vi "CVT Bool GetIndex.vi"(8 "error in (no error)":errorcluster, 11 "Tag Name":string) -> (0 "error out":errorcluster, 3 "Tag Index":i32)   [LabVIEW 2010]
uses:
  Current Value Table.lvlib
  DataTypes/Boolean_Get Index.vi
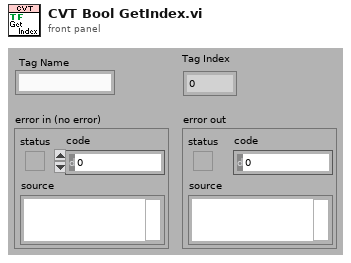
[diagram p1: front panel]
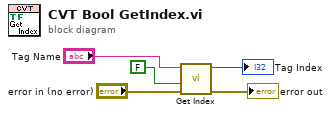
[diagram p0: block diagram]
diagram:
  n1 = call-poly "Get Index.vi"("error in (no error)"="error in (no error)", "Default"=FALSE ("Data Type"), "Tag Name"="Tag Name") -> ("error out"=→"error out":errorcluster, "Index"=→"Tag Index":i32)  [unwired: 7 in]
